vi "Get All Users.vi"(0 "User Manager Model in":refnum<class "User Manager Model.lvclass">, 11 "error in (no error)":errorcluster) -> (4 "User Manager Model out":refnum<class "User Manager Model.lvclass">, 15 "error out":errorcluster)   [LabVIEW 2020, in "User Manager Model.lvlib" / "User Manager Model.lvclass"]
uses:
  <vilib>/gpm_packages/@cs/User Manager App/User Manager Model/User Manager Model/User Manager Model.lvclass
  C:/Program Files/National Instruments/LabVIEW 2020/vi.lib/gpm_packages/@cs/mva-core/Source/IModel/IModel/IModel.lvclass
  <vilib>/gpm_packages/@cs/User Manager App/User Manager Model/Type Definitions/New User Information.ctl
  <vilib>/gpm_packages/@cs/User Manager App/User Manager Model/Type Definitions/Credentials.ctl
  <vilib>/gpm_packages/@cs/User Manager App/User Manager Model/Type Definitions/User Levels.ctl
  <vilib>/gpm_packages/@cs/User Manager App/User Manager Model/User Manager Model/User Manager Model.lvclass/User Manager Model.ctl
  <vilib>/gpm_packages/@cs/mva-core/Source/IObserver/IObserver/IObserver.lvclass/IObserver.ctl
  <vilib>/gpm_packages/@cs/mva-core/Source/IModel/IModel/IModel.lvclass/IModel.ctl
  <vilib>/gpm_packages/@cs/mva-core/Source/IMediator/PublishRequest/PublishRequest.lvclass/PublishRequest.ctl
  <vilib>/gpm_packages/@cs/mva-core/Source/IMediator/IMediator Messages/Publish Msg/Publish Msg.lvclass/Publish Msg.ctl
  <vilib>/gpm_packages/@cs/actor-framework-messages/Source/RoundTripMessage/RoundTripMessage.lvclass/RoundTripMessage.ctl
  <vilib>/ActorFramework/Message Enqueuer/Message Enqueuer.lvclass/Message Enqueuer.ctl
  <vilib>/gpm_packages/@cs/mva-core/Source/IMediator/IMediator Messages/Publish Msg/Send Pre-Addressed Publish.vi
  <vilib>/gpm_packages/@cs/mva-core/Source/IObserver/IObserver/Read Unique ID.vi
  <vilib>/gpm_packages/@cs/mva-core/Source/IMediator/PublishRequest/Pack Publish Request.vi
  <vilib>/gpm_packages/@cs/actor-framework-messages/Source/RoundTripMessage/Return Round-Trip Message.vi
  <vilib>/ActorFramework/Message Enqueuer/Enqueue.vi
  <vilib>/gpm_packages/@cs/mva-core/Source/IModel/IModel/IModel.lvclass
  C:/Program Files/National Instruments/LabVIEW 2020/vi.lib/gpm_packages/@cs/mva-core/Source/IObserver/IObserver/IObserver.lvclass
  <vilib>/gpm_packages/@cs/mva-core/Source/IMediator/IMediator Messages/Publish Msg/Publish Msg.lvclass
  C:/Program Files/National Instruments/LabVIEW 2020/vi.lib/gpm_packages/@cs/actor-framework-messages/Source/RoundTripMessage/RoundTripMessage.lvclass
  <vilib>/gpm_packages/@cs/actor-framework-messages/Source/RoundTripMessage/RoundTripMessage.lvclass
  C:/Program Files/National Instruments/LabVIEW 2020/vi.lib/ActorFramework/Message/Message.lvclass
  <vilib>/Utility/error.llb/Error Cluster From Error Code.vi
  <vilib>/ActorFramework/Message Priority Queue/Priority Enqueue.vi
  <vilib>/gpm_packages/@cs/mva-core/Source/IMediator/PublishRequest/PublishRequest.lvclass
  <vilib>/gpm_packages/@cs/user-manager/Source/User Configuration Manager Ref/By Ref.lvlib
  <vilib>/gpm_packages/@cs/User Manager App/User Manager Model/Type Definitions/User Manager Application Types.lvlib
panel:
  out "Array":T1[](array[typedef])
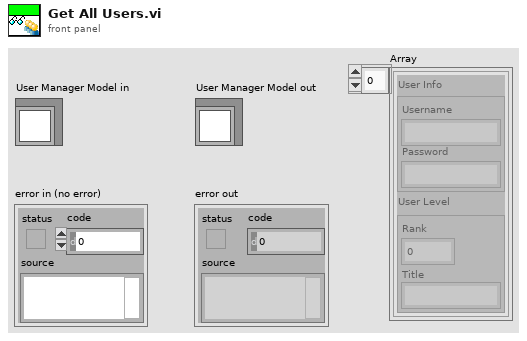
[diagram p1: front panel]
types:
  T1 = typedef "User Manager Application Types.lvlib/New User Information.ctl" = cluster{"User Info":T2, "User Level":T3}
  T2 = typedef "User Manager Application Types.lvlib/Credentials.ctl" = cluster{"Username":string, "Password":string}
  T3 = typedef "User Manager Application Types.lvlib/User Levels.ctl" = cluster{"Rank":i32, "Title":string}
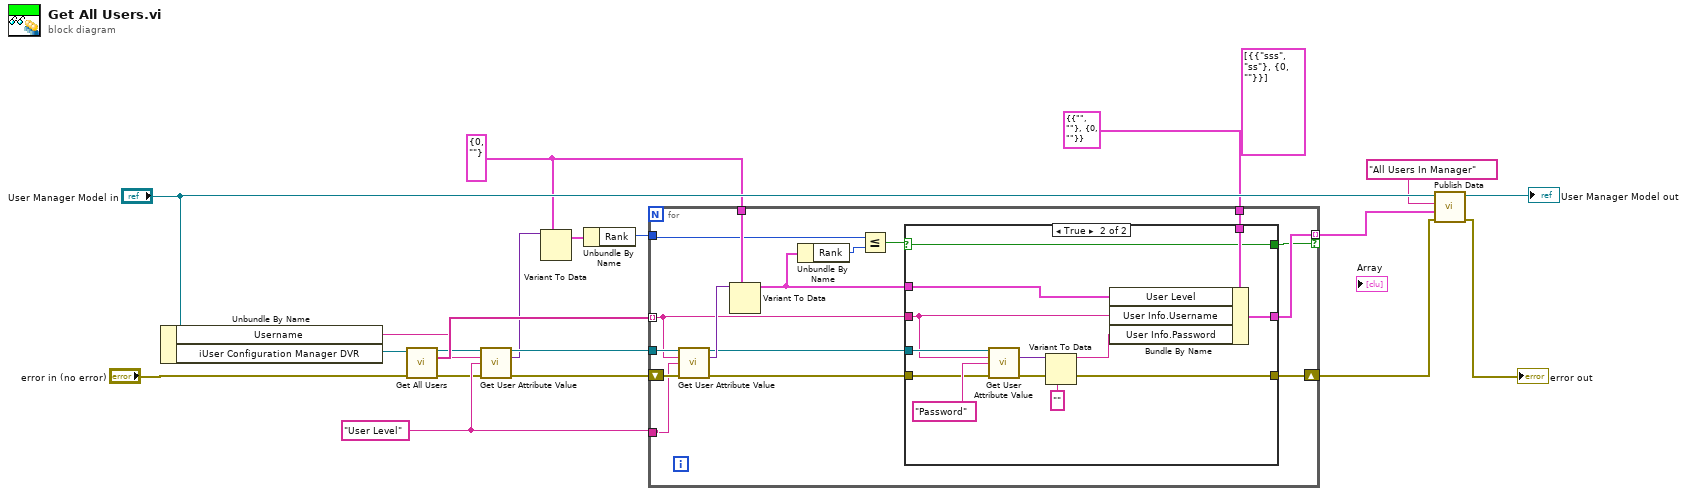
[diagram p0: block diagram]
diagram:
  (unwired) T1[] [{"User Info"={"Username"="sss", "Password"="ss"}, "User Level"={"Rank"=0, "Title"=""}}] ("New Uer Info")
  w6 = T3 {"Rank"=0, "Title"=""} ("User Level")
  w8 = "User Level" ("Attribute Name")
  n1 = Unbundle By Name("User Manager Model in") -> ("Username"=w9:string, "iUser Configuration Manager DVR"=w20:refnum<data-value>)
  n2 = call <vilib>:"Get All Users.vi"("iUser Configuration Manager DVR"=w20, "error in"="error in (no error)") -> ("dup iUser Configuration Manager DVR"=w13:refnum<data-value>, "Users"=w14:string[], "error out"=w3:errorcluster)  [unwired: 10 in, 1 out]
  n3 = call <vilib>:"Get User Attribute Value.vi"("iUser Configuration Manager DVR"=w13, "Username"=w9, "Attribute Name"=w8, "error in"=w3) -> ("dup iUser Configuration Manager DVR"=w10:refnum<data-value>, "Attribute Value"=w7:variant, "error out"=w2:errorcluster)  [unwired: 8 in, 1 out]
  n4 = Variant To Data(type=w6, Variant=w7) -> (data=w5:T3)  [unwired: 1 in, 1 out]
  n5 = Unbundle By Name(w5) -> ("Rank"=w4:i32)
  n6 = for {
    tunnel: w14 -> [w27] mode=indexing
    tunnel: T1 {"User Info"={"Username"="", "Password"=""}, "User Level"={"Rank"=0, "Title"=""}} ("New Uer Info") -> [w36]
    tunnel: [w35] -> w1 mode=indexing if=w25
    tunnel: w10 -> [w31]
    shift-right: [w24] -> w12
    shift-left: w2 -> [w28]
    tunnel: w8 -> [w21]
    tunnel: w6 -> [w33]
    tunnel: w4 -> [w32]
    n7 = call <vilib>:"Get User Attribute Value.vi"("iUser Configuration Manager DVR"=w31, "Username"=w27, "Attribute Name"=w21, "error in"=w28) -> ("dup iUser Configuration Manager DVR"=w30:refnum<data-value>, "Attribute Value"=w34:variant, "error out"=w26:errorcluster)  [unwired: 8 in, 1 out]
    n8 = Variant To Data(type=w33, Variant=w34) -> (data=w23:T3)  [unwired: 1 in, 1 out]
    n9 = Unbundle By Name(w23) -> ("Rank"=w22:i32)
    n10 = Less Or Equal?(x=w32, y=w22) -> (x <= y?=w29:bool)
    n11 = case shown="True" w29 {
      selector: w29 -> [w38 w44]
      tunnel: w36 -> [_ w50]
      tunnel: [_ w49] -> w35
      tunnel: w27 -> [_ w40]
      tunnel: w30 -> [_ w45]
      tunnel: w23 -> [_ w41]
      tunnel: [w38 w44] -> w25
      tunnel: w26 -> [w37 w43]
      tunnel: [w37 w42] -> w24
      frame False {
      }
      frame True {
        n12 = call <vilib>:"Get User Attribute Value.vi"("iUser Configuration Manager DVR"=w45, "Username"=w40, "Attribute Name"="Password", "error in"=w43) -> ("Attribute Value"=w46:variant, "error out"=w42:errorcluster)  [unwired: 8 in, 2 out]
        n13 = Variant To Data(type="", Variant=w46) -> (data=w39:string)  [unwired: 1 in, 1 out]
        n14 = Bundle By Name(cluster=w50, "User Level"=w41, "User Info.Username"=w40, "User Info.Password"=w39) -> (w49:T1)
      }
    }
  }
  n15 = call <vilib>:"Publish Data.vi"("error in (no error)"=w12, "Data to Publish"=w1, "Datum Name"="All Users In Manager", "IModel in"="User Manager Model in") -> ("error out"=→"error out":errorcluster, "IModel out"=→"User Manager Model out":refnum<class "User Manager Model.lvclass">)  [unwired: 6 in]
